vi "zad3.vi"() -> ()   [LabVIEW 2017]
panel:
  in  "Tryb awaryjny":bool
  in  "stop":bool
  out "Lampa Uliczna":cluster{"1":bool, "2":bool, "3":bool}
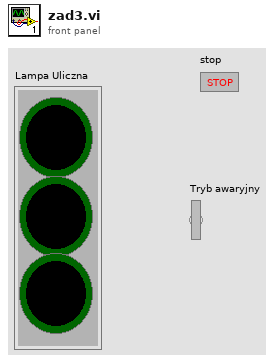
[diagram p1: front panel]
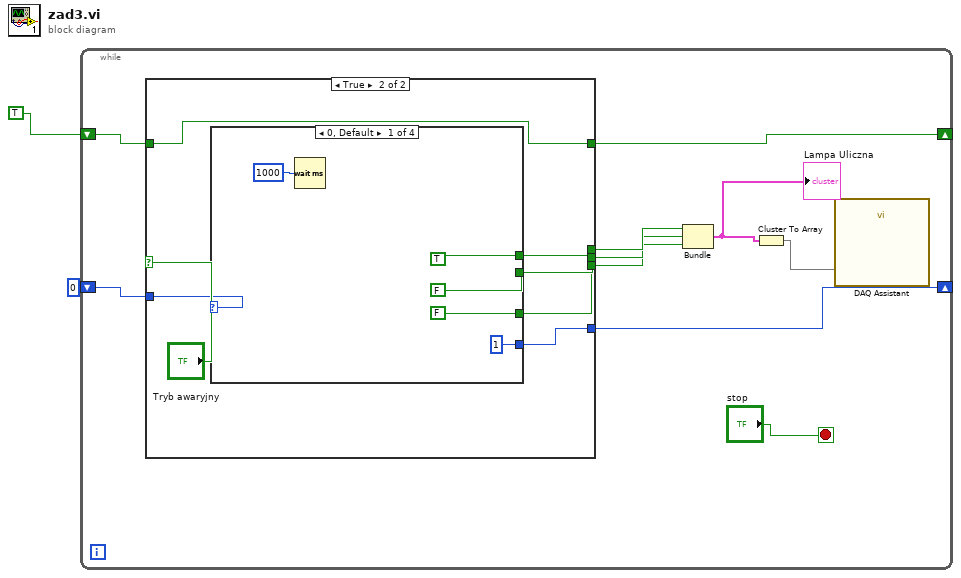
[diagram p0: block diagram]
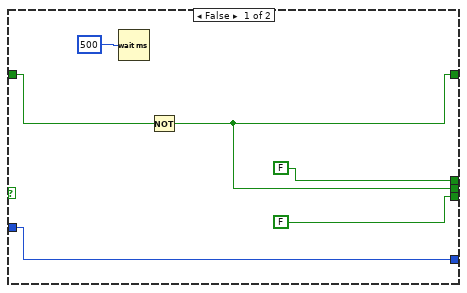
[diagram p2: hidden frame]
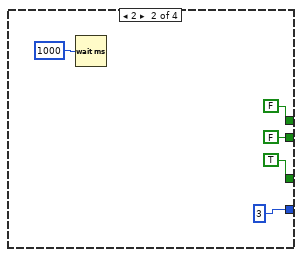
[diagram p3: hidden frame]
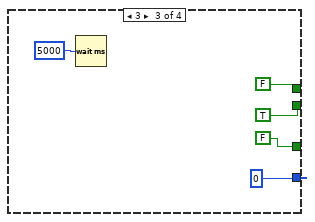
[diagram p4: hidden frame]
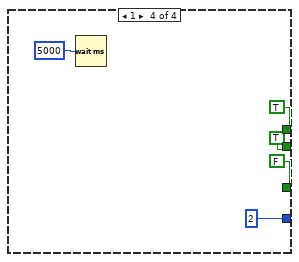
[diagram p5: hidden frame]
diagram:
  n1 = while {
    shift-right: [w11] -> _
    shift-left: 0 -> [w12]
    shift-right: [w8] -> _
    shift-left: TRUE ("2") -> [w9]
    stop <- "stop" stop-if-true
    n2 = case shown="True" "Tryb awaryjny" {
      tunnel: [w14 w25] -> w6
      tunnel: [FALSE ("3") w24] -> w5
      tunnel: [FALSE ("1") w23] -> w7
      tunnel: w12 -> [w17 w22]
      tunnel: [w17 w21] -> w11
      tunnel: [w14 w20] -> w8
      tunnel: w9 -> [w15 w20]
      frame False {
        n3 = Wait (ms)(milliseconds to wait=500) -> ()  [unwired: 1 out]
        n4 = Not(x=w15) -> (.not. x?=w14:bool)
      }
      frame True {
        n5 = case shown="0, Default" w22 {
          tunnel: [FALSE ("2") FALSE ("2") TRUE ("2") TRUE ("2")] -> w25
          tunnel: [FALSE ("3") TRUE ("3") FALSE ("3") FALSE ("3")] -> w24
          tunnel: [TRUE ("1") FALSE ("1") FALSE ("1") TRUE ("1")] -> w23
          tunnel: [1 3 0 2] -> w21
          frame 0, Default {
            n6 = Wait (ms)(milliseconds to wait=1000) -> ()  [unwired: 1 out]
          }
          frame 2 {
            n7 = Wait (ms)(milliseconds to wait=1000) -> ()  [unwired: 1 out]
          }
          frame 3 {
            n8 = Wait (ms)(milliseconds to wait=5000) -> ()  [unwired: 1 out]
          }
          frame 1 {
            n9 = Wait (ms)(milliseconds to wait=5000) -> ()  [unwired: 1 out]
          }
        }
      }
    }
    n10 = Bundle("1"=w7, "2"=w6, "3"=w5) -> (w4:cluster{"1":bool, "2":bool, "3":bool})  [unwired: 1 in]
    "Lampa Uliczna" <- w4
    n11 = Cluster To Array(cluster=w4) -> (array=w3:bool[])
    n12 = call "DAQ Assistant"("data"=w3) -> ()  [unwired: 17 in, 2 out]
  }
